vi "SaveallTraceAttribToMap.vi"(8 "error in (no error)":errorcluster, 10 "Map in":map{string, T1}(c390), 11 "XYGraph in":refnum<vi>) -> (0 "error out":errorcluster, 3 "Map out":map{string, T1}(c390))   [LabVIEW 2019]
uses:
  TraceData.ctl
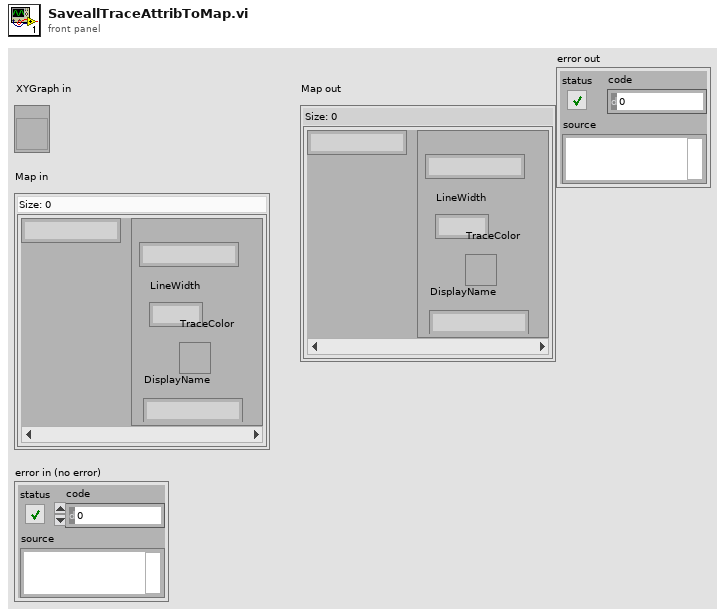
[diagram p1: front panel]
types:
  T1 = typedef "TraceData.ctl" = cluster{"Trace":string, "LineWidth":u8, "TraceColor":u32, "DisplayName":string}
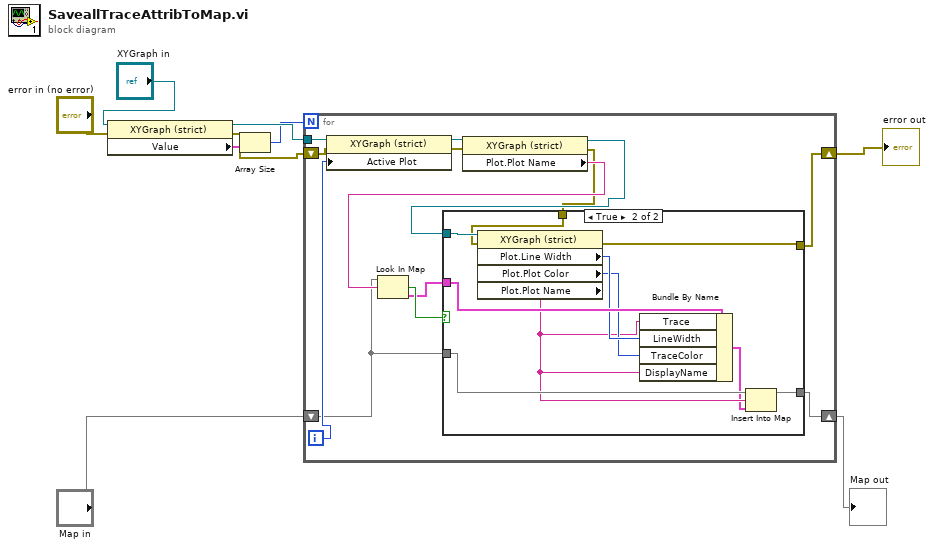
[diagram p0: block diagram]
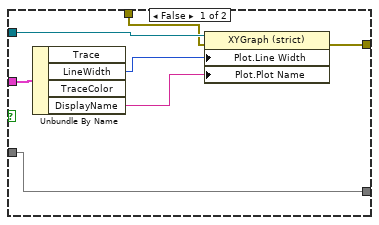
[diagram p2: hidden frame]
diagram:
  n1 = property class="XYGraph (strict)"(reference="XYGraph in", error in="error in (no error)") -> (reference out=w6:refnum<vi>, error out=w2:errorcluster, "Value"=w4:cluster{timestamp[], dbl[]}[])
  n2 = Array Size(array=w4) -> (size(s)=w5:i32)
  n3 = for {
    N: w5 -> [_]
    tunnel: w6 -> [w22]
    shift-right: [w13] -> w9
    shift-left: "Map in" -> [w14]
    shift-right: [w10] -> w1
    shift-left: w2 -> [w12]
    i -> [w21]
    n4 = property class="XYGraph (strict)"(reference=w22, error in=w12, "Active Plot"=w21) -> (reference out=w20:refnum<vi>, error out=w19:errorcluster)
    n5 = property class="XYGraph (strict)"(reference=w20, error in=w19) -> (reference out=w15:refnum<vi>, error out=w11:errorcluster, "Plot.Plot Name"=w18:string)
    n6 = Look In Map(map=w14, key=w18) -> (key not found?=w17:bool, value=w16:T1)  [unwired: 1 in]
    n7 = case shown="True" w17 {
      tunnel: w16 -> [w29 w38]
      tunnel: w15 -> [w28 w39]
      tunnel: w14 -> [w25 w35]
      tunnel: [w25 w32] -> w13
      tunnel: w11 -> [w24 w31]
      tunnel: [w23 w30] -> w10
      frame False {
        n8 = Unbundle By Name(w29) -> ("LineWidth"=w27:u8, "DisplayName"=w26:string)  [unwired: 2 out]
        n9 = property class="XYGraph (strict)"(reference=w28, error in=w24, "Plot.Line Width"=w27, "Plot.Plot Name"=w26) -> (error out=w23:errorcluster)  [unwired: 1 out]
      }
      frame True {
        n10 = property class="XYGraph (strict)"(reference=w39, error in=w31) -> (error out=w30:errorcluster, "Plot.Line Width"=w37:u8, "Plot.Plot Color"=w36:u32, "Plot.Plot Name"=w34:string)  [unwired: 1 out]
        n11 = Bundle By Name(cluster=w38, "Trace"=w34, "LineWidth"=w37, "TraceColor"=w36, "DisplayName"=w34) -> (w33:T1)
        n12 = Insert Into Map(map in=w35, key=w34, value=w33) -> (map out=w32:map{string, T1})  [unwired: 2 out]
      }
    }
  }
  "Map out" <- w9
  "error out" <- w1
